vi "read reverse power W.vi"(0 "VISA resource name":refnum<visa-resource-name>="GPIB0::12::INSTR", 1 "error in (no error)":errorcluster) -> (2 "VISA resource name out":refnum<visa-resource-name>, 3 "Reverse Power (W)":dbl[unit], 4 "error out":errorcluster)   [LabVIEW 2009]
uses:
  MicrowaveAmp.lvlib
panel:
  out "read buffer":string
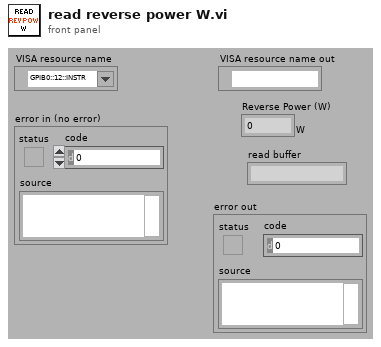
[diagram p1: front panel]
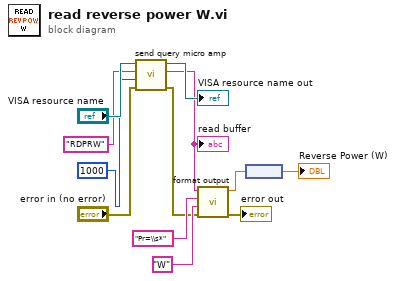
[diagram p0: block diagram]
diagram:
  n1 = call "send query micro amp.vi"("error in (no error)"="error in (no error)", "Bytes Count"=u32 1000 ("bytes to read (1000) 2"), "write buffer"="RDPRW" ("write buffer 2"), "VISA resource name"="VISA resource name") -> ("error out"=w5:errorcluster, "read buffer"=w1:string, "VISA resource name out"=→"VISA resource name out":refnum<visa-resource-name>)  [unwired: 5 in]
  "read buffer" <- w1
  n2 = call "format output.vi"("error in (no error)"=w5, "Search for String"="W" ("search string"), "Regular Expression"="Pr=\\s*" ("search string"), "Input String"=w1) -> ("error out"=→"error out":errorcluster, "Output"=w8:dbl)  [unwired: 6 in]
  n3 = node(w8) -> (→"Reverse Power (W)":dbl[unit])
